vi "Main.vi"() -> ()   [LabVIEW 2018]
uses:
  <vilib>/myRIO/Instrument Drivers/Onboard IO/AI/typedefs/AI Reference.ctl
  <vilib>/myRIO/Common/Instrument Driver Framework/Utilities/typedefs/myRIO Generic Hardware Reference.ctl
  <vilib>/myRIO/Common/Instrument Driver Framework/Utilities/typedefs/Hardware Version Enum.ctl
  <vilib>/myRIO/Common/Instrument Driver Framework/Utilities/typedefs/myRIO v1.0 Reference.ctl
  <vilib>/myRIO/Common/Instrument Driver Framework/Utilities/typedefs/Generic FPGA Reference.ctl
  <vilib>/myRIO/Common/Instrument Driver Framework/myRIO v1.0/AI/typedefs/AI Channels List.ctl
  <vilib>/myRIO/Common/Instrument Driver Framework/myRIO v1.0/AI/typedefs/AI Channels Enum.ctl
  <vilib>/myRIO/Common/Instrument Driver Framework/Utilities/typedefs/Analog Scaling Constants List.ctl
  <vilib>/myRIO/Common/Instrument Driver Framework/Utilities/typedefs/Analog Scaling Constants.ctl
  <vilib>/userdefined/High Color/nirio_resource_hc.ctl
  <vilib>/myRIO/Common/Instrument Driver Framework/myRIO v1.0/AI/vis/myRIO v1.1 Open AI.vi
  <vilib>/myRIO/Common/Instrument Driver Framework/Utilities/vis/Validate Channels.vi
  <vilib>/myRIO/Common/Instrument Driver Framework/myRIO v1.0/AI/vis/myRIO v1.0 Reserve AI.vi
  <vilib>/myRIO/Common/Instrument Driver Framework/myRIO v1.0/AI/vis/myRIO v1.0 Close AI.vi
  <vilib>/myRIO/Common/Instrument Driver Framework/myRIO v1.0/AI/vis/myRIO v1.0 Build MUX Configuration AI.vi
  <vilib>/myRIO/Common/Instrument Driver Framework/myRIO v1.0/Resource Manager/vis/myRIO v1.0 Reserve Channel List.vi
  <vilib>/myRIO/Common/Instrument Driver Framework/myRIO v1.0/AI/vis/myRIO v1.0 Unreserve AI.vi
  <vilib>/myRIO/Common/Instrument Driver Framework/myRIO v1.0/Resource Manager/vis/myRIO v1.0 Reserve Channel.vi
  <vilib>/myRIO/Common/Instrument Driver Framework/myRIO v1.0/Resource Manager/vis/myRIO v1.0 Unreserve Channel.vi
  <vilib>/myRIO/Common/Instrument Driver Framework/myRIO v1.0/Resource Manager/vis/myRIO v1.0 Unreserve Channel List.vi
  <vilib>/myRIO/Common/Instrument Driver Framework/myRIO v1.0/Resource Manager/vis/myRIO v1.0 Build Mutex Name.vi
  <vilib>/Utility/VariantDataType/GetNumericInfo.vi
  <vilib>/Utility/error.llb/Error Cluster From Error Code.vi
  <vilib>/myRIO/Common/Instrument Driver Framework/myRIO v1.0/myRIO v1.1 Open.vi
  <vilib>/myRIO/Common/Instrument Driver Framework/myRIO v1.0/AI/vis/myRIO v1.0 Get Scaling Constants AI.vi
  <vilib>/myRIO/Common/Instrument Driver Framework/Utilities/vis/IO Manager.vi
  <vilib>/myRIO/Common/Instrument Driver Framework/Utilities/vis/Configuration Manager.vi
  <vilib>/myRIO/Common/Instrument Driver Framework/myRIO v1.0/myRIO v1.0 Close.vi
  <vilib>/myRIO/Common/Instrument Driver Framework/myRIO v1.0/AI/vis/myRIO v1.0 Read AI.vi
  <vilib>/express/express analysis/Spectral/Block/exnSpectralBlock spectral measurements power poly.vi
  <vilib>/express/express analysis/Spectral/Block/exnSpectralBlock spectral measurements power DDT.vi
  <vilib>/myRIO/Instrument Drivers/Onboard IO/AI/vis/myRIO AI Open.xnode
  <vilib>/express/express analysis/Spectral/XNode/ExpressSpectralMeasurementsBlockNode.xnode
  <vilib>/myRIO/Instrument Drivers/Onboard IO/AI/AI.lvlib
panel:
  out "EEG":cluster{dbl[], dbl[]}(graph)
  in  "Measure":bool caption="Blank Button"
  in  "Save":bool
  out "Filtered Signal":dynamicdata(graph)
  out "Spectrum":dynamicdata(graph)
  in  "Stop":bool
  in  "Start":bool
  out "Enum":T1(ring)
  out "Error Out":errorcluster
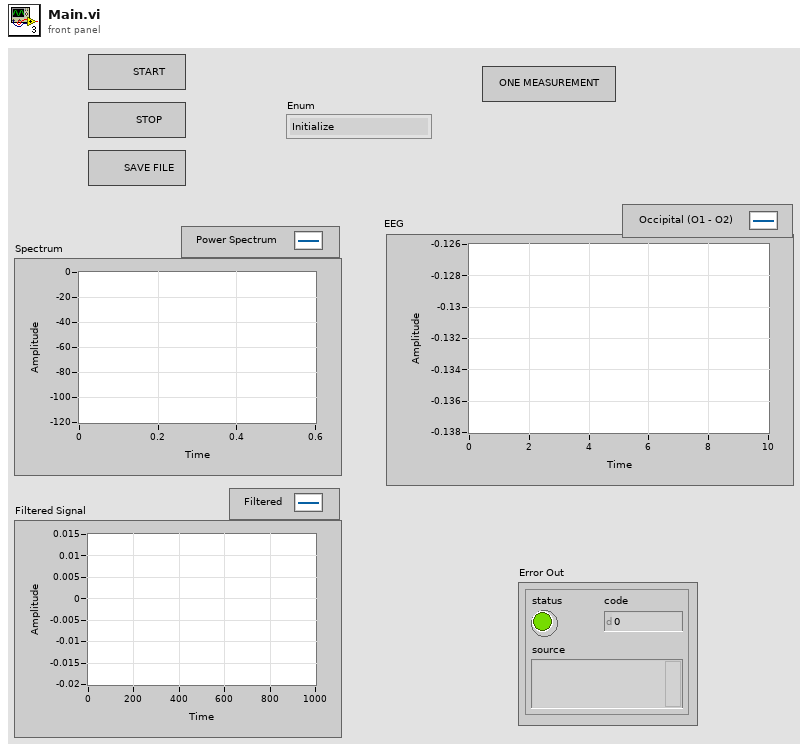
[diagram p1: front panel]
types:
  T1 = enum16{"Initialize", "Standby", "Record Data", "Filter Signal", "Save to File", "Stop"}
  T2 = typedef "nirio_resource_hc.ctl" = tag
  T3 = typedef "Hardware Version Enum.ctl" = enum16{"Unknown", "myRIO-1900", "myRIO-1950", "roboRIO", "NI ELVIS RIO CM", "ELVIS III"}
  T4 = cluster{"averaging mode":u16, "weighting mode":u16, "number of averages":u32}
  T5 = cluster{"dB On (F)":bool, "unwrap phase (F)":bool, "convert to degree (F)":bool}
  T6 = typedef "AI.lvlib/AI Reference.ctl" = cluster{"myRIO Reference":T7, "AI Channels List":T10, "AI Scaling Constants List":T12}
  T7 = typedef "myRIO Generic Hardware Reference.ctl" = cluster{"myRIO Model":T3, "myRIO Hardware Reference":T8}
  T8 = typedef "myRIO v1.0 Reference.ctl" = cluster{"Generic FPGA Reference":T9, "Allow multiple opens":bool}
  T9 = typedef "Generic FPGA Reference.ctl" = refnum<k20>
  T10 = typedef "AI Channels List.ctl" = T11[]
  T11 = typedef "AI Channels Enum.ctl" = enum16{"Not Connected", "AudioIn/Left", "AudioIn/Right", "C/AI0", "C/AI1", "A/AI0", "A/AI1", "A/AI2", "A/AI3", "A/AI4", "A/AI5", "A/AI6", "A/AI7", "B/AI0", "B/AI1", "B/AI2", "B/AI3", "B/AI4", "B/AI5", "B/AI6", "B/AI7", "AI/AI0", "AI/AI1", "AI/AI2", "AI/AI3", "A/AI0 (DIFF)", "A/AI1 (DIFF)", "A/AI2 (DIFF)", "A/AI3 (DIFF)", "B/AI0 (DIFF)", "B/AI1 (DIFF)", "B/AI2 (DIFF)", "B/AI3 (DIFF)"}
  T12 = typedef "Analog Scaling Constants List.ctl" = T13[]
  T13 = typedef "Analog Scaling Constants.ctl" = cluster{"LSB Weight (Volts)":dbl, "Offset (Volts)":dbl, "Signed?":bool}
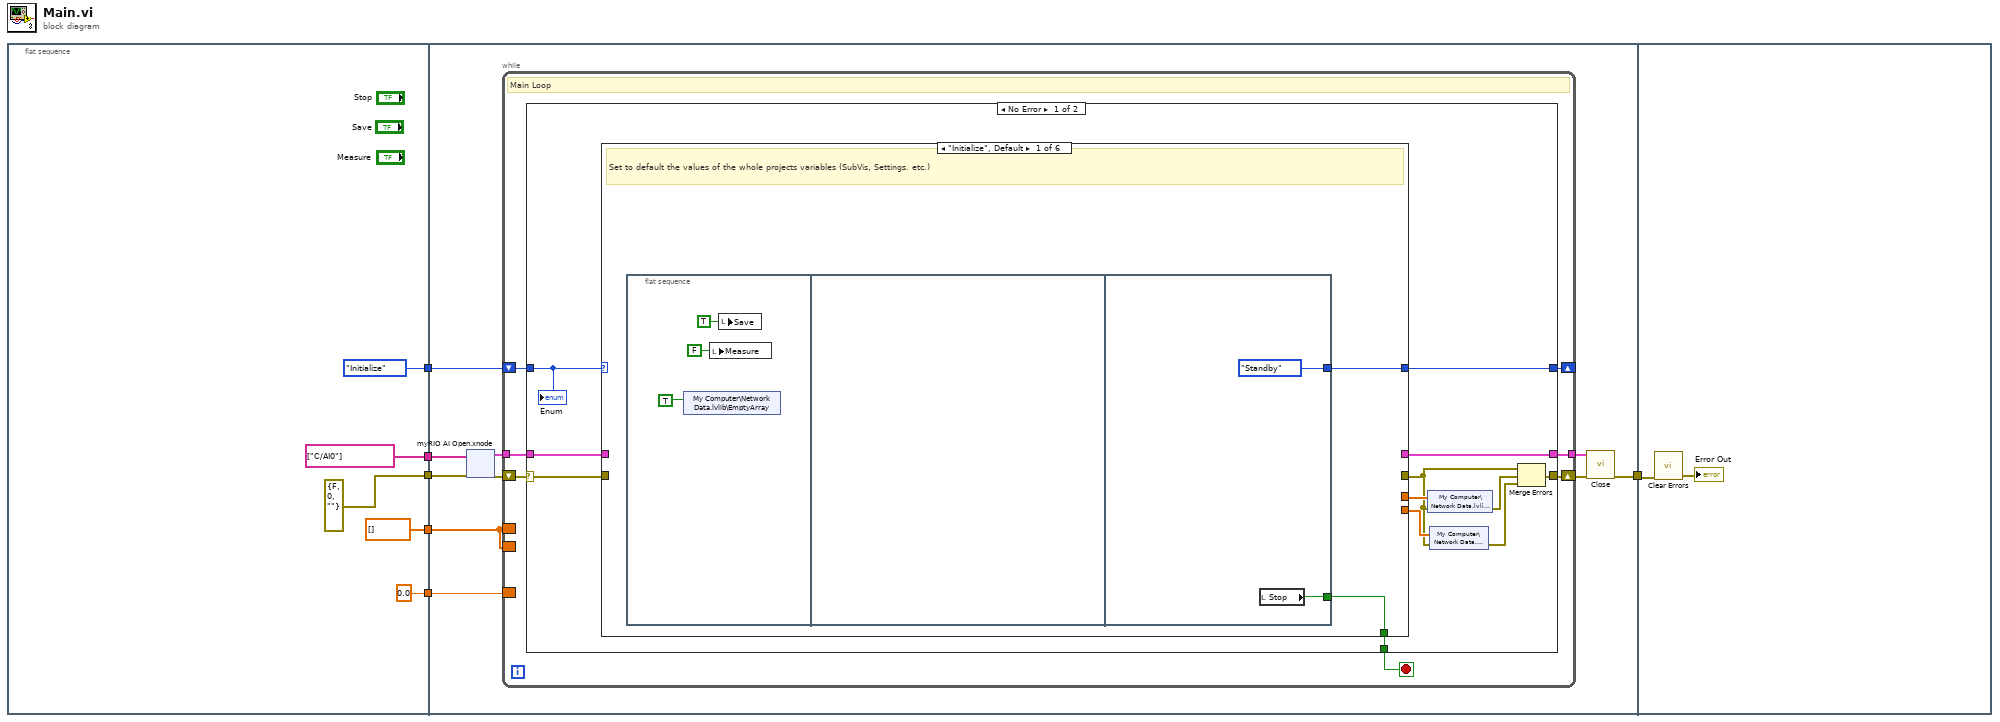
[diagram p0: block diagram]
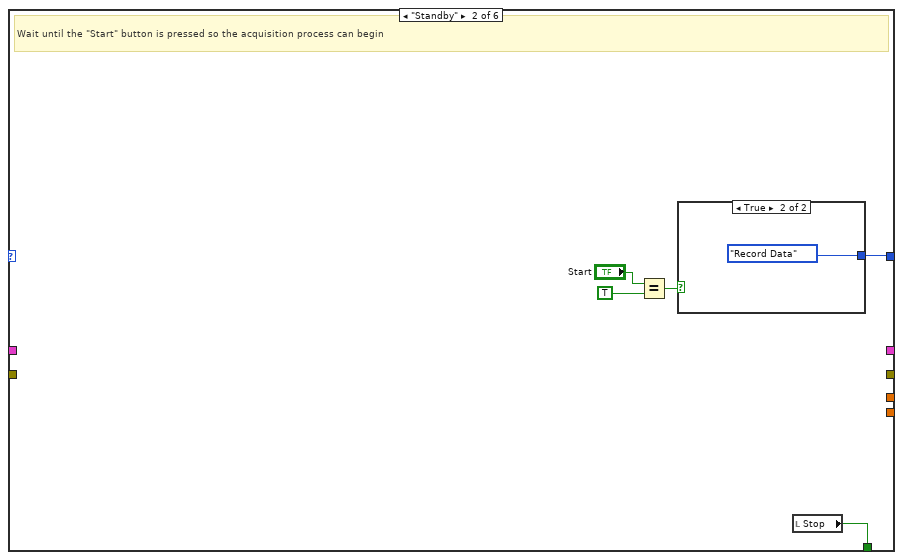
[diagram p2: hidden frame]
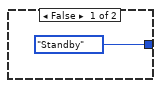
[diagram p3: hidden frame]
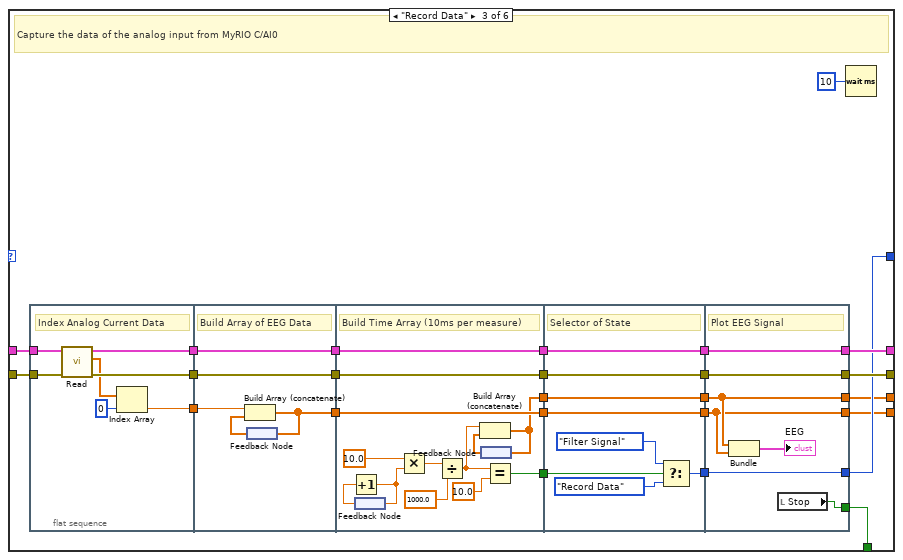
[diagram p4: hidden frame]
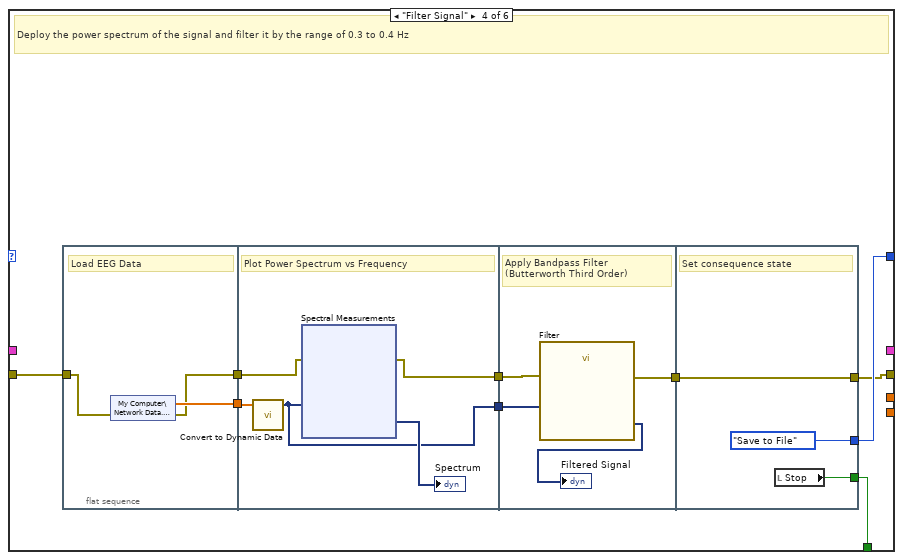
[diagram p5: hidden frame]
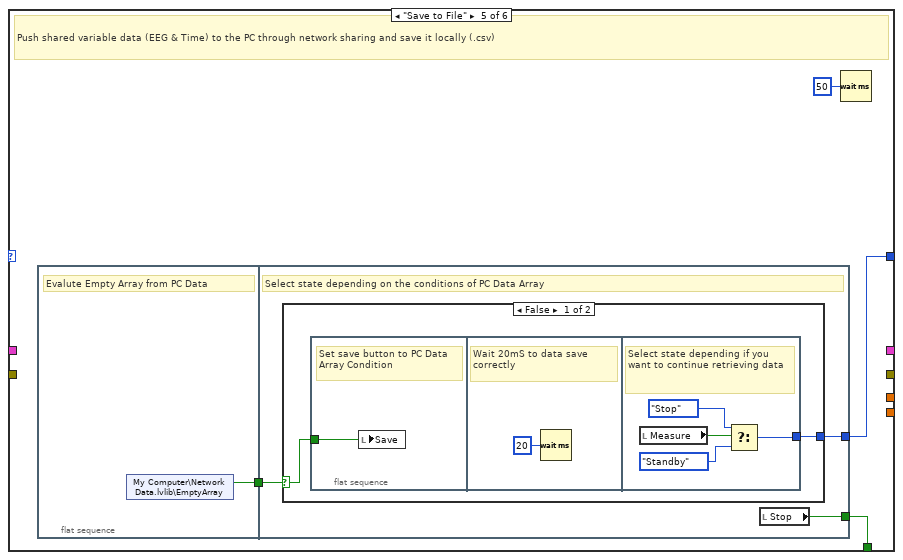
[diagram p6: hidden frame]
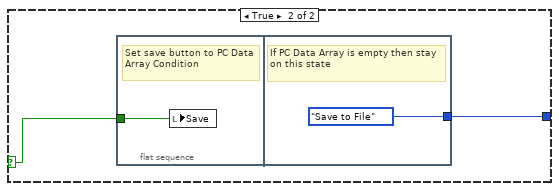
[diagram p7: hidden frame]
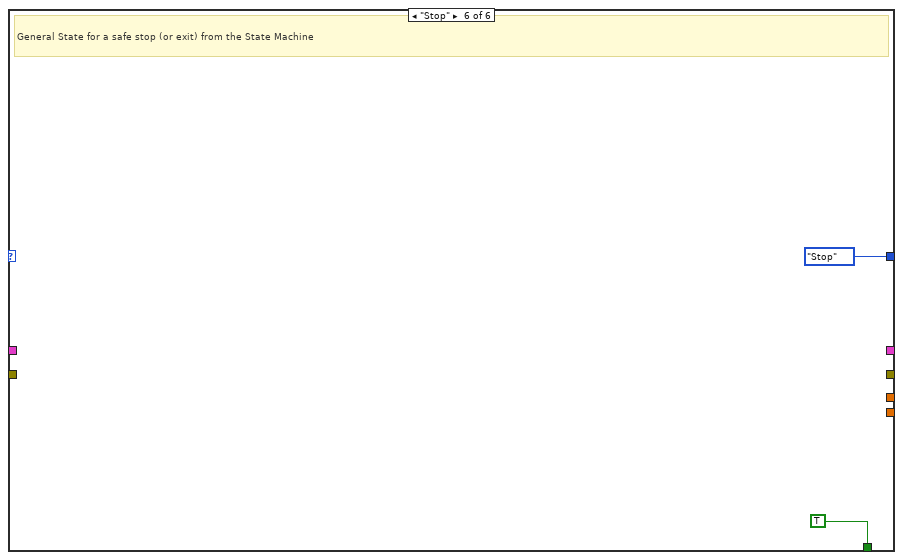
[diagram p8: hidden frame]
diagram:
  n1 = flat-sequence {
    tunnel: [T1."Initialize"] -> w6
    tunnel: [tag[] ["C/AI0"] ("Channel Names")] -> w5
    tunnel: [errorcluster {"status"=FALSE, "code"=0, "source"=""} ("error constant")] -> w4
    tunnel: [0.0] -> w2
    tunnel: [dbl[] []] -> w1
    tunnel: w6 -> [w21]
    tunnel: w5 -> [w20]
    tunnel: w4 -> [w17]
    tunnel: [w14] -> w3
    tunnel: w2 -> [w13]
    tunnel: w1 -> [w12]
    tunnel: w3 -> [w197]
    frame #0 {
    }
    frame #1 {
      n2 = xnode "myRIO AI Open.xnode"("error in (no error)"=w17, "Channel Names"=w20) -> ("error out"=w19:errorcluster, "AI Ref Out"=w18:T6)  [unwired: 1 in]
      n3 = while {
        shift-right: [w45] -> _
        shift-left: w21 -> [w46]
        tunnel: w18 -> [w44]
        tunnel: [w43] -> w16
        border: w13 -> [_]
        border: w12 -> [_]
        border: w12 -> [_]
        shift-right: [w41] -> w15
        shift-left: w19 -> [w40]
        stop <- w42 stop-if-true
        # "Main Loop"
        n4 = case shown="No Error" w40 {
          selector: w40 -> [w47 w195]
          tunnel: w46 -> [w58 w193]
          tunnel: [w57 w193] -> w45
          tunnel: w44 -> [w56 w194]
          tunnel: [w55 w194] -> w43
          tunnel: [w52 _] -> w42
          tunnel: [w51 w195] -> w41
          frame No Error {
            n5 = case shown="\"Initialize\", Default" w58 {
              tunnel: [w60 w70 w85 w145 w172 T1."Stop"] -> w57
              tunnel: w56 -> [_ _ w97 _ _ _]
              tunnel: w47 -> [_ _ w96 w142 _ _]
              tunnel: [_ _ w95 _ _ _] -> w55
              tunnel: [_ _ w94 w140 _ _] -> w50
              tunnel: [_ _ w80 _ _ _] -> w54
              tunnel: [_ _ w79 _ _ _] -> w53
              tunnel: [w59 w66 w78 w138 w171 TRUE] -> w52
              frame "Initialize", Default {
                # "Set to default the values of the whole projects variables (SubVis, Settings. etc.)"
                n6 = flat-sequence {
                  tunnel: [T1."Standby"] -> w60
                  tunnel: [w64] -> w59
                  frame #0 {
                    n7 = shared-variable "My Computer\\Network Data.lvlib\\EmptyArray"(TRUE) -> ()  [unwired: 1 in, 1 out]
                    n8 = local write "Measure"(FALSE ("Measure")) -> ()
                    n9 = local write "Save"(TRUE ("Save")) -> ()
                  }
                  frame #1 {
                  }
                  frame #2 {
                    n10 = local read "Stop"() -> (w64:bool)
                  }
                }
              }
              frame "Standby" {
                # "Wait until the \"Start\" button is pressed so the acquisition process can begin"
                n11 = Equal?(x="Start", y=TRUE) -> (x = y?=w69:bool)
                n12 = case shown="True" w69 {
                  tunnel: [T1."Standby" T1."Record Data"] -> w70
                  frame False {
                  }
                  frame True {
                  }
                }
                n13 = local read "Stop"() -> (w66:bool)
              }
              frame "Record Data" {
                # "Capture the data of the analog input from MyRIO C/AI0"
                n14 = flat-sequence {
                  tunnel: w97 -> [w104]
                  tunnel: w96 -> [w103]
                  tunnel: [w102] -> w93
                  tunnel: [w101] -> w92
                  tunnel: [w98] -> w89
                  tunnel: w93 -> [w109]
                  tunnel: w92 -> [w108]
                  tunnel: [w109] -> w91
                  tunnel: [w108] -> w90
                  tunnel: w89 -> [w107]
                  tunnel: [w105] -> w82
                  tunnel: w91 -> [w122]
                  tunnel: w90 -> [w121]
                  tunnel: [w122] -> w88
                  tunnel: [w121] -> w87
                  tunnel: [w114] -> w86
                  tunnel: [w111] -> w83
                  tunnel: w82 -> [w111]
                  tunnel: [w110] -> w81
                  tunnel: w88 -> [w130]
                  tunnel: w87 -> [w129]
                  tunnel: w86 -> [w127]
                  tunnel: w83 -> [w124]
                  tunnel: w81 -> [w123]
                  tunnel: [w130] -> w77
                  tunnel: [w129] -> w76
                  tunnel: [w128] -> w75
                  tunnel: [w124] -> w74
                  tunnel: [w123] -> w73
                  tunnel: [w134] -> w78
                  tunnel: [w133] -> w80
                  tunnel: [w132] -> w79
                  tunnel: [w135] -> w85
                  tunnel: [w136] -> w94
                  tunnel: [w137] -> w95
                  tunnel: w77 -> [w137]
                  tunnel: w76 -> [w136]
                  tunnel: w75 -> [w135]
                  tunnel: w74 -> [w132]
                  tunnel: w73 -> [w133]
                  frame #0 {
                    # "Index Analog Current Data"
                    n15 = call <vilib>:"Read.vi"("error in (no error)"=w103, "AI Ref In"=w104) -> ("error out"=w101:errorcluster, "Values"=w100:dbl[], "AI Ref Out"=w102:T6)  [unwired: 7 in]
                    n16 = Index Array(array=w100, index=0) -> (element=w98:dbl)
                  }
                  frame #1 {
                    # "Build Array of EEG Data"
                    n17 = feedback #1() -> (w106:dbl[])
                    n18 = Build Array (concatenate)(w107, w106) -> (w105:dbl[])
                    n19 = feedback-in #1(w105) -> ()
                  }
                  frame #2 {
                    # "Build Time Array (10ms per measure)"
                    n20 = feedback #2() -> (w120:dbl)
                    n21 = Increment(x=w120) -> (x+1=w119:dbl)
                    n22 = feedback-in #2(w119) -> ()
                    n23 = Multiply(x=10.0, y=w119) -> (x*y=w117:dbl)
                    n24 = Divide(x=w117, y=1000.0) -> (x/y=w113:dbl)
                    n25 = feedback #3() -> (w112:dbl[])
                    n26 = Build Array (concatenate)(w113, w112) -> (w110:dbl[])
                    n27 = feedback-in #3(w110) -> ()
                    n28 = Equal?(x=w113, y=10.0) -> (x = y?=w114:bool)
                  }
                  frame #3 {
                    # "Selector of State"
                    n29 = Select(t=T1."Filter Signal", s=w127, f=T1."Record Data") -> (s? t:f=w128:T1)
                  }
                  frame #4 {
                    # "Plot EEG Signal"
                    n30 = Bundle(w133, w132) -> (→"EEG":cluster{dbl[], dbl[]})  [unwired: 1 in]
                    n31 = local read "Stop"() -> (w134:bool)
                  }
                }
                n32 = Wait (ms)(milliseconds to wait=u32 10) -> ()  [unwired: 1 out]
              }
              frame "Filter Signal" {
                # "Deploy the power spectrum of the signal and filter it by the range of 0.3 to 0.4 Hz"
                n33 = flat-sequence {
                  tunnel: [w149] -> w146
                  tunnel: [w147] -> w143
                  tunnel: w142 -> [w148]
                  tunnel: w146 -> [w154]
                  tunnel: [w152] -> w144
                  tunnel: w143 -> [w151]
                  tunnel: [w150] -> w141
                  tunnel: w144 -> [w166]
                  tunnel: w141 -> [w165]
                  tunnel: [w164] -> w139
                  tunnel: [T1."Save to File"] -> w145
                  tunnel: [w169] -> w140
                  tunnel: w139 -> [w169]
                  tunnel: [w168] -> w138
                  frame #0 {
                    # "Load EEG Data"
                    n34 = shared-variable "My Computer\\Network Data.lvlib\\EEG"(error in=w148) -> (w149:dbl[], error out=w147:errorcluster)
                  }
                  frame #1 {
                    # "Plot Power Spectrum vs Frequency"
                    n35 = call "Convert to Dynamic Data"("Array"=w154) -> ("Dynamic Data Type"=w152:dynamicdata)  [unwired: 3 in]
                    n36 = xnode "Spectral Measurements"("Signals"=w152, "error in (no error)"=w151) -> ("Power Spectrum"=→"Spectrum":dynamicdata, "error out"=w150:errorcluster)
                  }
                  frame #2 {
                    # "Apply Bandpass Filter\n(Butterworth Third Order)"
                    n37 = call "Filter"("error in (no error)"=w165, "Signal"=w166) -> ("error out"=w164:errorcluster, "Filtered Signal"=→"Filtered Signal":dynamicdata)  [unwired: 8 in]
                  }
                  frame #3 {
                    # "Set consequence state"
                    n38 = local read "Stop"() -> (w168:bool)
                  }
                }
              }
              frame "Save to File" {
                # "Push shared variable data (EEG & Time) to the PC through network sharing and save it locally (.csv)"
                n39 = flat-sequence {
                  tunnel: [w175] -> w173
                  tunnel: w173 -> [w177]
                  tunnel: [w178] -> w172
                  tunnel: [w176] -> w171
                  frame #0 {
                    # "Evalute Empty Array from PC Data"
                    n40 = shared-variable "My Computer\\Network Data.lvlib\\EmptyArray"() -> (w175:bool)  [unwired: 1 in, 1 out]
                  }
                  frame #1 {
                    # "Select state depending on the conditions of PC Data Array"
                    n41 = case shown="False" w177 {
                      selector: w177 -> [w179 w187]
                      tunnel: [w180 w188] -> w178
                      frame False {
                        n42 = flat-sequence {
                          tunnel: w179 -> [w181]
                          tunnel: [w183] -> w180
                          frame #0 {
                            # "Set save button to PC Data Array Condition"
                            n43 = local write "Save"(w181) -> ()
                          }
                          frame #1 {
                            # "Wait 20mS to data save correctly"
                            n44 = Wait (ms)(milliseconds to wait=u32 20) -> ()  [unwired: 1 out]
                          }
                          frame #2 {
                            # "Select state depending if you want to continue retrieving data"
                            n45 = local read "Measure"() -> (w186:bool)
                            n46 = Select(t=T1."Stop", s=w186, f=T1."Standby") -> (s? t:f=w183:T1)
                          }
                        }
                      }
                      frame True {
                        n47 = flat-sequence {
                          tunnel: w187 -> [w189]
                          tunnel: [T1."Save to File"] -> w188
                          frame #0 {
                            # "Set save button to PC Data Array Condition"
                            n48 = local write "Save"(w189) -> ()
                          }
                          frame #1 {
                            # "If PC Data Array is empty then stay on this state"
                          }
                        }
                      }
                    }
                    n49 = local read "Stop"() -> (w176:bool)
                  }
                }
                n50 = Wait (ms)(milliseconds to wait=u32 50) -> ()  [unwired: 1 out]
              }
              frame "Stop" {
                # "General State for a safe stop (or exit) from the State Machine"
              }
            }
            n51 = shared-variable "My Computer\\Network Data.lvlib\\Time"(w54, error in=w50) -> (error out=w49:errorcluster)
            n52 = shared-variable "My Computer\\Network Data.lvlib\\EEG"(w53, error in=w50) -> (error out=w48:errorcluster)
            n53 = Merge Errors(w50, w49, w48) -> (w51:errorcluster)
            "Enum" <- w58
          }
          frame Error {
          }
        }
      }
      n54 = call <vilib>:"Close.vi"("error in (no error)"=w15, "AI Ref In"=w16) -> ("error out"=w14:errorcluster)  [unwired: 9 in]
    }
    frame #2 {
      n55 = call <vilib>:"Clear Errors.vi"("error in (no error)"=w197) -> ("error out"=→"Error Out":errorcluster)  [unwired: 5 in, 1 out]
    }
  }
